vi "Split bytes.vi"(8 "error in":errorcluster, 9 "End index":i32, 10 "Start index":i32, 11 "bytes in":u8[](array[numeric])) -> (0 "error out":errorcluster, 2 "selected bytes":u8[](array[numeric]), 3 "remaining bytes":u8[](array[numeric]), 4 "before bytes":u8[](array[numeric]))   [LabVIEW 2020, in "MessagePack.lvlib" / "MessagePack.lvclass"]
uses:
  MessagePack.lvclass
  <vilib>/Utility/error.llb/Error Cluster From Error Code.vi
  <vilib>/ErrorRing/Error Ring.xnode
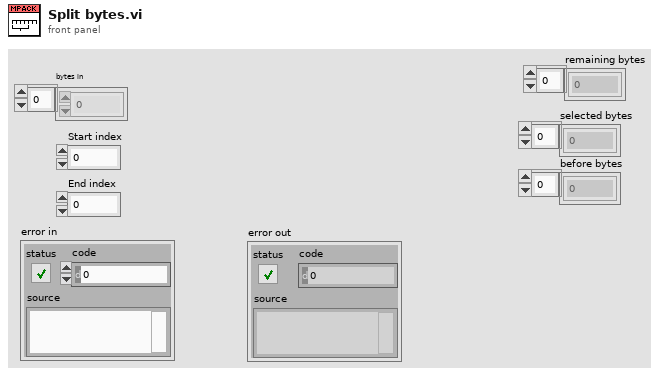
[diagram p1: front panel]
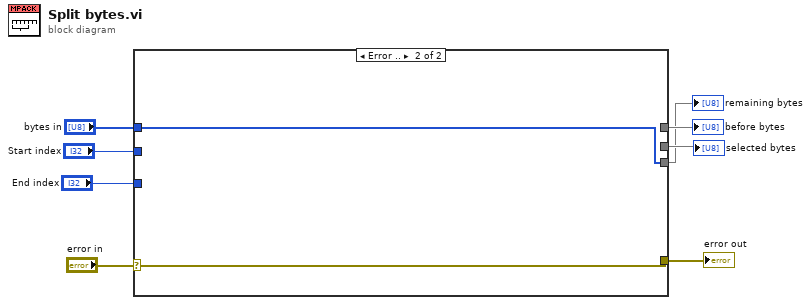
[diagram p0: block diagram]
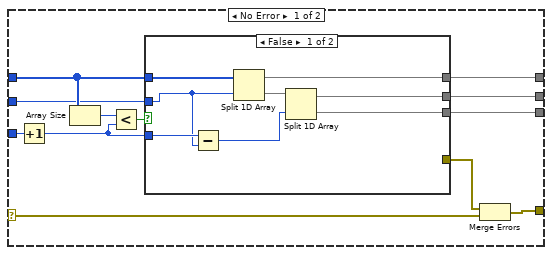
[diagram p2: hidden frame]
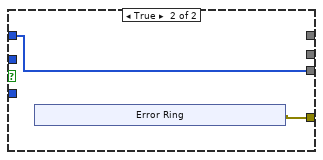
[diagram p3: hidden frame]
diagram:
  n1 = case shown="Error .." "error in" {
    selector: "error in" -> [w18 w36]
    tunnel: [w16 w36] -> w7
    tunnel: "Start index" -> [w14 _]
    tunnel: "bytes in" -> [w15 w35]
    tunnel: "End index" -> [w12 _]
    tunnel: [w13 _] -> w3
    tunnel: [w10 _] -> w2
    tunnel: [w9 w35] -> w1
    frame No Error {
      n2 = Increment(x=w12) -> (x+1=w11:i32)
      n3 = Array Size(array=w15) -> (size(s)=w20:i32)
      n4 = Less?(x=w20, y=w11) -> (x < y?=w19:bool)
      n5 = case shown="False" w19 {
        tunnel: [_ w30] -> w17
        tunnel: w15 -> [w28 w29]
        tunnel: w14 -> [w24 _]
        tunnel: [w27 _] -> w13
        tunnel: w11 -> [w25 _]
        tunnel: [w22 _] -> w10
        tunnel: [w21 w29] -> w9
        frame False {
          n6 = Subtract(x=w25, y=w24) -> (x-y=w23:i32)
          n7 = Split 1D Array(array=w28, index=w24) -> (first subarray=w27:u8[], second subarray=w26:u8[])
          n8 = Split 1D Array(array=w26, index=w23) -> (first subarray=w22:u8[], second subarray=w21:u8[])
        }
        frame True {
          n9 = xnode "Error Ring"() -> ("error out"=w30:errorcluster)
        }
      }
      n10 = Merge Errors(w17, w18) -> (w16:errorcluster)
    }
    frame Error {
    }
  }
  "error out" <- w7
  "selected bytes" <- w2
  "remaining bytes" <- w1
  "before bytes" <- w3
